vi "Actor Core.vi"(8 "error in":errorcluster, 11 "Configurator Actor:Configuration UI Actor in":refnum<class "Configuration UI Actor.lvclass">) -> (0 "error out":errorcluster, 3 "Configurator Actor:Configuration UI Actor out":refnum<class "Actor.lvclass">)   [LabVIEW 2023, in "Configuration UI Actor.lvlib" / "Configuration UI Actor.lvclass"]
doc: "(<B>Filename</B>: Actor Framework.lvlib:Actor.lvclass:Actor Core.vi)\n\nReceives messages to the actor, reacts to them, and initiates any error handling that may shut the actor down.\n\nDescendant classes may override this VI to append parallel tasks for the actor to complete while it handles messages. Overrides use the Call Parent Method node."
uses:
  Configuration UI Actor.lvclass
  <vilib>/ActorFramework/Actor/Actor.lvclass
  Database/Database UI/Database UI.lvclass
  HAL GOOP4/Scope/Scope Simulated/Configurations/Fetch Waveforms CFG/Fetch Waveforms CFG.lvclass
  HAL GOOP4/Scope/Virtual Scopes/Virt Voltage Reader/Virt Voltage Reader.lvclass
  HAL GOOP4/FGen/FGen Simulated/Configurations/Generate DC CFG/Generate DC CFG.lvclass
  HAL GOOP4/FGen/Virtual FGens/Virt Voltage Generator/Virt Voltage Generator.lvclass
  HAL GOOP4/FGen/Virtual FGens/Virt Waveform Generator/Virt Std Waveform Generator.lvclass
  gitlab/imponator-series-actor/Imponator Series Actor/Imponator Series UI Actor/Imponator Series UI Actor.lvclass
  HAL GOOP4/DIO/Virtual DIO/Virt PWM Fixed Freq Generator/Virt DAQmx Fixed Freq PWM Generator.lvclass
  HAL GOOP4/DIO/DIO DAQmx Simulated CFGs/DO DAQmx PWM Fixed Freq CFG/DO DAQmx Fixed Freq PWM CFG.lvclass
  HAL GOOP4/DIO/DO DAQmx Fixed Freq PWM CFG/DO DAQmx Fixed Freq PWM CFG.lvclass
  gitlab/imponator-series-actor/Imponator Series Actor/Tasks/Boot Up/Valves and Fans/Task Boot Up Valves and Fans.lvclass
  gitlab/imponator-series-actor/Imponator Series Actor/Tasks/Stack/Task Stack.lvclass
  HAL GOOP4/Thermometer/Thermometer DAQmx RTD Cont CFG/Thermometer DAQmx RTD Cont CFG.lvclass
  HAL GOOP4/Virt Instr Target/Virt Instr Target.lvclass
  Configuration UI Actor.lvclass/Configuration UI Actor.ctl
  <vilib>/ActorFramework/Actor/Actor.lvclass/Actor.ctl
  <vilib>/ActorFramework/Message Enqueuer/Message Enqueuer.lvclass/Message Enqueuer.ctl
  <vilib>/ActorFramework/Message Enqueuer/Init from Existing Queue.vi
  <vilib>/ActorFramework/Message Enqueuer/Enqueue.vi
  <vilib>/MGI/Panel Manager/Panel/Panel/Subpanel/Subpanel.lvclass
  <vilib>/ActorFramework/Stop Msg/Stop Msg.lvclass
  Configuration UI Actor Messages/Launch Series Msg/Launch Series Msg.lvclass
  <vilib>/MGI/Panel Manager/Panel/Panel/Subpanel/Subpanel.vi
  <vilib>/Utility/LVClass/Get LV Class Name.vi
  <resource>/AFDebug/Generate Trace for Message.vi
  <vilib>/ActorFramework/Message Priority Queue/Priority Enqueue.vi
  <vilib>/ActorFramework/Message Enqueuer/Message Enqueuer.lvclass
  <vilib>/MGI/Panel Manager/Panel Actor/Panel Actor/Panel Actor.lvclass
  Messages/Set Instr CFG_Msg/Set Instr CFG_Msg.lvclass
  <vilib>/MGI/Panel Manager/Panel/Panel.lvlib
  C:/Program Files/National Instruments/LabVIEW 2023/vi.lib/MGI/Panel Manager/Panel Actor/Panel Actor/Panel Actor.lvclass
  C:/Program Files/National Instruments/LabVIEW 2023/vi.lib/ActorFramework/Actor/Actor.lvclass
  D:/git/HAL/Configurator/Configuration UI Actor/Configuration UI Actor.lvclass
  D:/git/HAL/Configurator/IConfiguration UI Actor/IConfiguration UI Actor/IConfiguration UI Actor.lvclass
  D:/git/HAL/Database/Database UI/Database UI.lvclass
  D:/git/HAL/Database/IDatabase UI/IDatabase UI/IDatabase UI.lvclass
  C:/Program Files/National Instruments/LabVIEW 2023/vi.lib/MGI/Panel Manager/Panel/Panel/Panel.lvclass
  C:/Program Files/National Instruments/LabVIEW 2023/vi.lib/MGI/Panel Manager/Panel/Panel/Subpanel/Subpanel.lvclass
panel:
  in  "Launch Series":bool
  out "Series Valid":cluster{"JSON":bool, "CFG":bool}
  in  "Series CFG":string
  out "Virt Valid":cluster{"JSON":bool, "CFG":bool}
  out "Instr Valid":cluster{"JSON":bool, "CFG":bool}
  in  "Instr CFG Selector":string(combo)
  in  "Instr CFG":string
  in  "Virt Instrs CFG":string
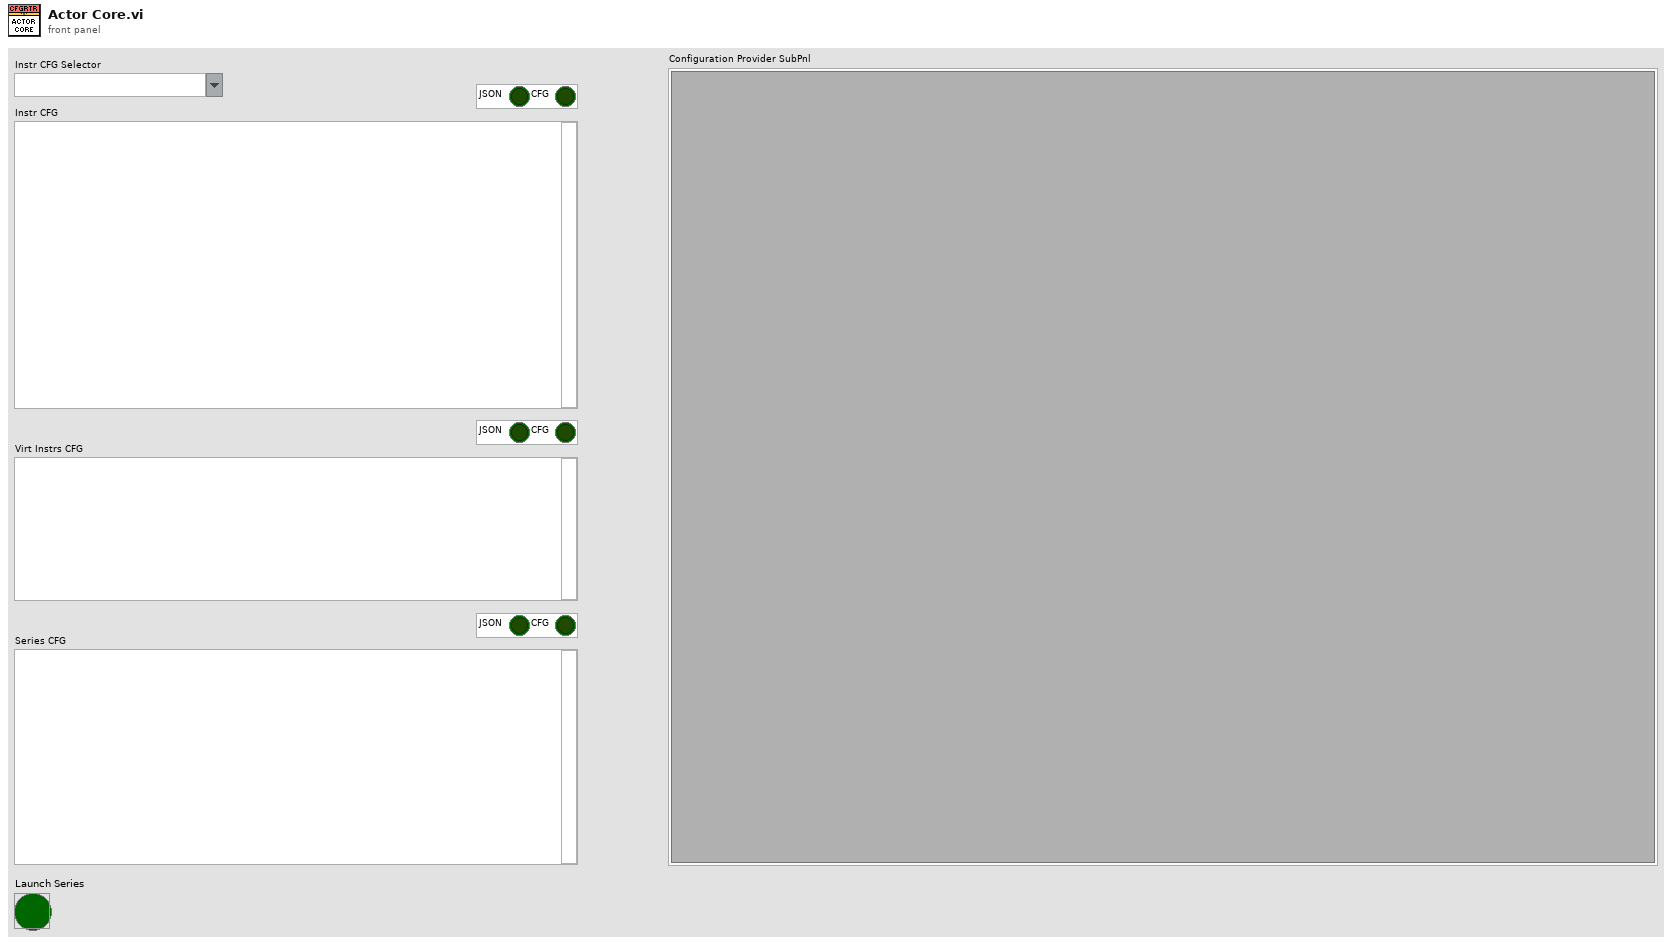
[diagram p1: front panel]
types:
  T1 = cluster{"Stop":refnum<user-event>, "Instr Valid":refnum<user-event>, "Virt Valid":refnum<user-event>, "Series Valid":refnum<user-event>}
  T2 = cluster{"Pnl Actor":refnum<event-registration>, "Event Registration Refnum":refnum<event-registration>}
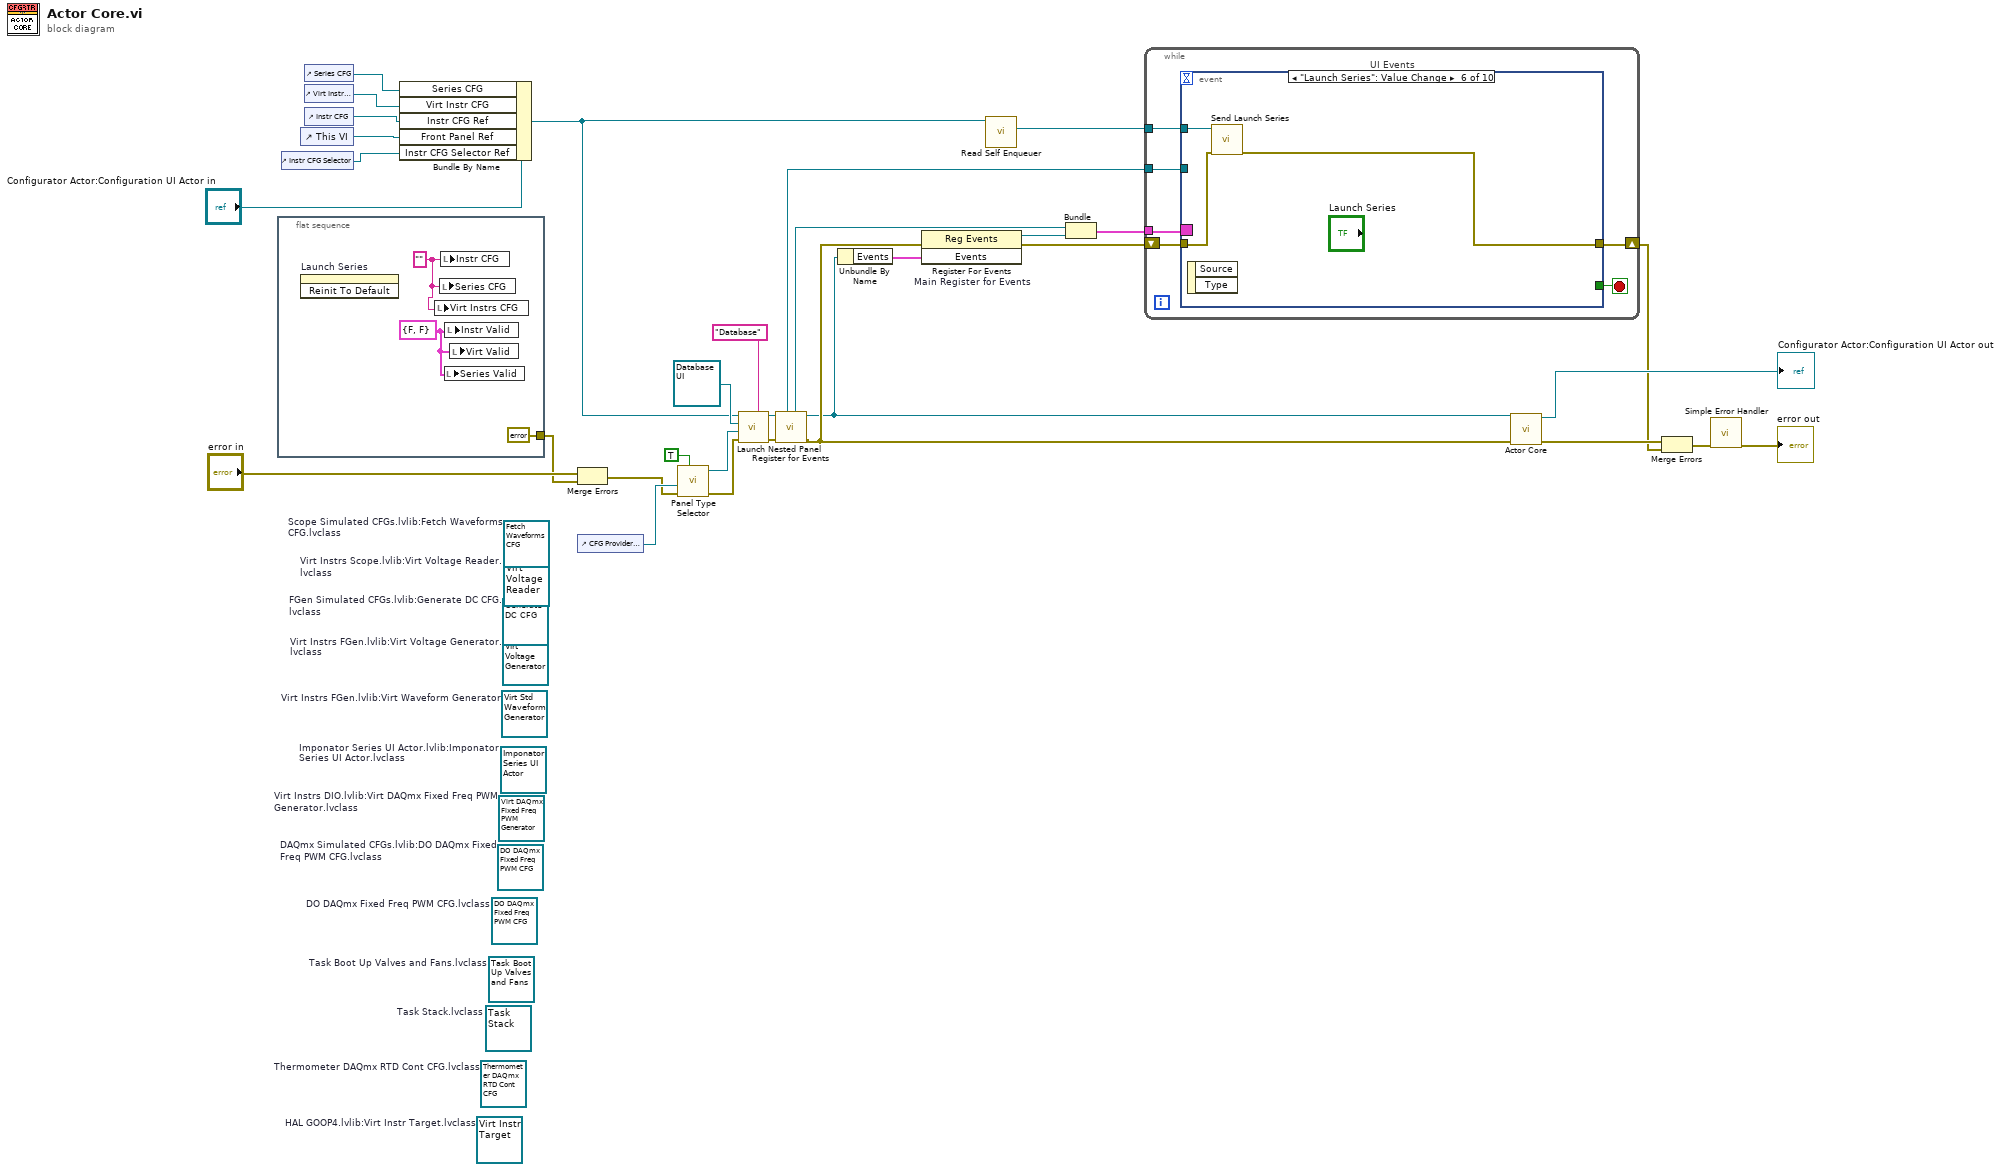
[diagram p0: block diagram]
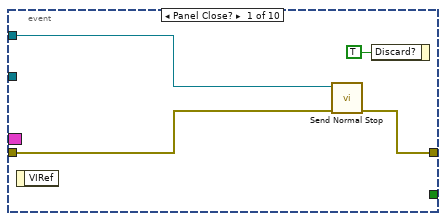
[diagram p2: hidden frame]
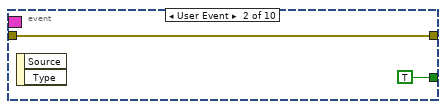
[diagram p3: hidden frame]
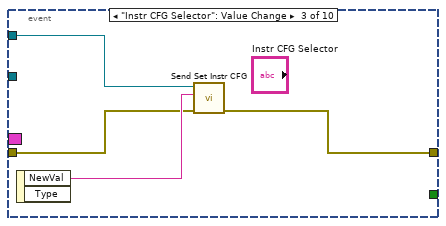
[diagram p4: hidden frame]
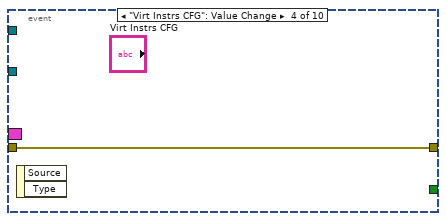
[diagram p5: hidden frame]
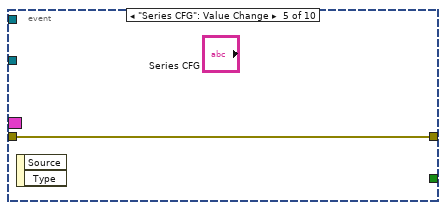
[diagram p6: hidden frame]
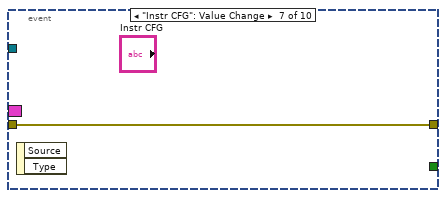
[diagram p7: hidden frame]
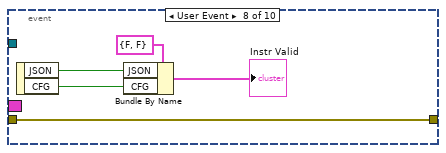
[diagram p8: hidden frame]
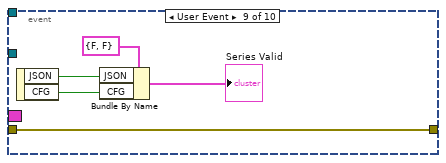
[diagram p9: hidden frame]
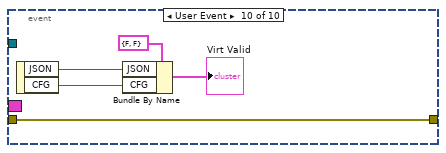
[diagram p10: hidden frame]
diagram:
  (unwired) refnum<class "Virt Instr Target.lvclass"> refnum  # HAL GOOP4.lvlib:Virt Instr Target.lvclass
  (unwired) refnum<class "Thermometer DAQmx RTD Cont CFG.lvclass"> refnum  # Thermometer DAQmx RTD Cont CFG.lvclass
  (unwired) refnum<class "Task Stack.lvclass"> refnum  # Task Stack.lvclass
  (unwired) refnum<class "Task Boot Up Valves and Fans.lvclass"> refnum  # Task Boot Up Valves and Fans.lvclass
  (unwired) refnum<class "DO DAQmx Fixed Freq PWM CFG.lvclass"> refnum  # DO DAQmx Fixed Freq PWM CFG.lvclass
  (unwired) refnum<class "DO DAQmx Fixed Freq PWM CFG.lvclass"> refnum  # DAQmx Simulated CFGs.lvlib:DO DAQmx Fixed Freq PWM CFG.lvclass
  (unwired) refnum<class "Virt DAQmx Fixed Freq PWM Generator.lvclass"> refnum  # Virt Instrs DIO.lvlib:Virt DAQmx Fixed Freq PWM Generator.lvclass
  (unwired) refnum<class "Imponator Series UI Actor.lvclass"> refnum  # Imponator Series UI Actor.lvlib:Imponator Series UI Actor.lvclass
  (unwired) refnum<class "Virt Std Waveform Generator.lvclass"> refnum  # Virt Instrs FGen.lvlib:Virt Waveform Generator
  (unwired) refnum<class "Virt Voltage Generator.lvclass"> refnum  # Virt Instrs FGen.lvlib:Virt Voltage Generator.lvclass
  (unwired) refnum<class "Generate DC CFG.lvclass"> refnum  # FGen Simulated CFGs.lvlib:Generate DC CFG.lvclass
  (unwired) refnum<class "Virt Voltage Reader.lvclass"> refnum  # Virt Instrs Scope.lvlib:Virt Voltage Reader.lvclass
  (unwired) refnum<class "Fetch Waveforms CFG.lvclass"> refnum  # Scope Simulated CFGs.lvlib:Fetch Waveforms CFG.lvclass
  n1 = flat-sequence {
    tunnel: [errorcluster {"status"=FALSE, "code"=0, "source"=""} ("error in (no error)")] -> w1
    frame #0 {
      w34 = cluster{"JSON":bool, "CFG":bool} {"JSON"=FALSE, "CFG"=FALSE} ("Instr Valid")
      w35 = "" ("Instr CFG")
      n2 = invoke on="Launch Series" class="Bool" method="Reinit To Default"() -> ()  [unwired: 3 in, 3 out]
      n3 = local write "Virt Instrs CFG"(w35) -> ()
      n4 = local write "Series CFG"(w35) -> ()
      n5 = local write "Instr CFG"(w35) -> ()
      n6 = local write "Series Valid"(w34) -> ()
      n7 = local write "Instr Valid"(w34) -> ()
      n8 = local write "Virt Valid"(w34) -> ()
    }
  }
  n9 = control-ref of="Instr CFG Selector"() -> (w18:refnum<vi>)
  n10 = control-ref of="This VI"() -> (w29:refnum<vi>)
  n11 = control-ref of="Series CFG"() -> (w15:refnum<vi>)
  n12 = control-ref of="Virt Instrs CFG"() -> (w27:refnum<vi>)
  n13 = control-ref of="Instr CFG"() -> (w28:refnum<vi>)
  n14 = Bundle By Name(cluster="Configurator Actor:Configuration UI Actor in", "Series CFG"=w15, "Virt Instr CFG"=w27, "Instr CFG Ref"=w28, "Front Panel Ref"=w29, "Instr CFG Selector Ref"=w18) -> (w6:refnum<class "Configuration UI Actor.lvclass">)
  n15 = Merge Errors("error in", w1) -> (w2:errorcluster)
  n16 = control-ref of="CFG Provider SubPnl"() -> (w7:refnum<vi>)
  n17 = call-poly <vilib>:"Panel Type Selector.vi"("Autoshow? (T)"=TRUE, "Error In"=w2, "Sub Panel"=w7) -> ("Error Out"=w3:errorcluster, "Subpanel Out"=w8:refnum<class "Subpanel.lvclass">)  [unwired: 7 in]
  n18 = call <vilib>:"Launch Nested Panel.vi"("Debug Alias"="Database", "error in (no error)"=w3, "Panel"=w8, "Nested Panel Actor"=refnum<class "Database UI.lvclass"> refnum ("Database UI.lvlib:Database UI.lvclass"), "Panel Actor in"=w6) -> ("error out"=w9:errorcluster, "Panel Actor out"=w10:refnum<class "Configuration UI Actor.lvclass">)  [unwired: 3 in, 2 out]
  n19 = call <vilib>:"Register for Events.vi"("Error In"=w9, "Panel Actor in"=w10) -> ("Error Out"=w23:errorcluster, "Panel Actor out"=w17:refnum<class "Configuration UI Actor.lvclass">, "Pnl Actor"=w20:refnum<event-registration>, "Self Enqueuer"=w11:refnum<class "Message Enqueuer.lvclass">)  [unwired: 6 in]
  n20 = Unbundle By Name(w17) -> ("Events"=w26:T1)
  n21 = register-events "Main Register for Events"(error in=w23, w26) -> (reference out=w21:refnum<event-registration>, error out=w25:errorcluster)  [unwired: 1 in]
  n22 = call <vilib>:"Read Self Enqueuer.vi"("Actor"=w6) -> ("Self Enqueuer"=w30:refnum<class "Message Enqueuer.lvclass">)  [unwired: 10 in]
  n23 = Bundle("Pnl Actor"=w20, "Event Registration Refnum"=w21) -> (w22:T2)  [unwired: 1 in]
  n24 = while {
    tunnel: w22 -> [w41]
    tunnel: w30 -> [w39]
    shift-right: [w37] -> w19
    shift-left: w25 -> [w38]
    tunnel: w11 -> [w36]
    stop <- w40 stop-if-true
    n25 = event "UI Events" shown="[5] \"Launch Series\": Value Change" {
      selector: w41 -> [_ _ _ _ _ _ _ _ _ _]
      dyn-events: _ -> [_ _ _ _ _ _ _ _ _ _]
      timeout: _ -> [_ _ _ _ _ _ _ _ _ _]
      tunnel: [_ TRUE _ _ _ _ _ _ _ _] -> w40
      tunnel: w39 -> [w44 _ w51 _ _ w56 _ _ _ _]
      tunnel: w38 -> [w43 w46 w49 w52 w53 w55 w57 w58 w63 w68]
      tunnel: [w42 w46 w48 w52 w53 w54 w57 w58 w63 w68] -> w37
      tunnel: w36 -> [_ _ _ _ _ _ _ _ _ _]
      event Panel Close? {
        n26 = event-data() -> ()  [unwired: 1 in, 1 out]
        n27 = call <vilib>:"Send Normal Stop.vi"("error in (no error)"=w43, "Message Enqueuer"=w44) -> ("error out"=w42:errorcluster)  [unwired: 9 in]
        n28 = event-data("Discard?"=TRUE) -> ()  [unwired: 1 in, 1 out]
      }
      event User Event {
        n29 = event-data() -> ()  [unwired: 1 in, 2 out]
      }
      event "Instr CFG Selector": Value Change {
        n30 = event-data() -> ("NewVal"=w50:string)  [unwired: 1 in, 1 out]
        n31 = call "Send Set Instr CFG.vi"("error in (no error)"=w49, "Instr Ident"=w50, "Message Enqueuer"=w51) -> ("error out"=w48:errorcluster)  [unwired: 7 in, 1 out]
      }
      event "Virt Instrs CFG": Value Change {
        n32 = event-data() -> ()  [unwired: 1 in, 2 out]
      }
      event "Series CFG": Value Change {
        n33 = event-data() -> ()  [unwired: 1 in, 2 out]
      }
      event "Launch Series": Value Change {
        n34 = event-data() -> ()  [unwired: 1 in, 2 out]
        n35 = call "Send Launch Series.vi"("error in (no error)"=w55, "Message Enqueuer"=w56) -> ("error out"=w54:errorcluster)  [unwired: 8 in, 1 out]
      }
      event "Instr CFG": Value Change {
        n36 = event-data() -> ()  [unwired: 1 in, 2 out]
      }
      event User Event {
        n37 = event-data() -> ("JSON"=w60:bool, "CFG"=w59:bool)  [unwired: 1 in]
        n38 = Bundle By Name(cluster=cluster{"JSON":bool, "CFG":bool} {"JSON"=FALSE, "CFG"=FALSE} ("Instr Valid"), "JSON"=w60, "CFG"=w59) -> (→"Instr Valid":cluster{"JSON":bool, "CFG":bool})
      }
      event User Event {
        n39 = event-data() -> ("JSON"=w66:bool, "CFG"=w65:bool)  [unwired: 1 in]
        n40 = Bundle By Name(cluster=cluster{"CFG":bool, "JSON":bool} {"CFG"=FALSE, "JSON"=FALSE}, "JSON"=w66, "CFG"=w65) -> (→"Series Valid":cluster{"CFG":bool, "JSON":bool})
      }
      event User Event {
        n41 = event-data() -> ("JSON"=w70:bool, "CFG"=w69:bool)  [unwired: 1 in]
        n42 = Bundle By Name(cluster=cluster{"JSON":bool, "CFG":bool} {"JSON"=FALSE, "CFG"=FALSE} ("Virt Valid"), "JSON"=w70, "CFG"=w69) -> (→"Virt Valid":cluster{"JSON":bool, "CFG":bool})
      }
    }
  }
  n43 = call-parent "Actor Core.vi"("error in"=w23, "Panel Actor in"=w17) -> ("error out"=w32:errorcluster, "Actor out"=→"Configurator Actor:Configuration UI Actor out":refnum<class "Actor.lvclass">)  [unwired: 8 in]
  n44 = Merge Errors(w32, w19) -> (w24:errorcluster)
  n45 = call <vilib>:"Simple Error Handler.vi"("error in (no error)"=w24) -> ("error out"=→"error out":errorcluster)  [unwired: 4 in, 4 out]
